vi "ParameterCtl.vi"(8 "error in":errorcluster caption="错误输入（无错误）", 9 "设备索引":u16(ring) caption="索引" items=["0", "1", "2", "3", "4", "5", "6", "7"], 11 "参数输入":T3={"帧ID1"=0, "等待延时"=0, "间隔延时"=0, "总时间"=0, "总次数"=0, "发送数据1"="", "接收数据1"="", "发送数据2"="", "接收数据2"="", "CAN盒类型"=3, "帧ID2"=0, "同步启动个数"=8, "模式"=enum."整体", "Baud"=12} {"Baud" items=["250k bps"=10, "10k bps"=2, "5k bps"=1, "50k bps"=5, "40k bps"=4, "20k bps"=3, "80k bps"=6, "100k bps"=7, "125k bps"=8, "200k bps"=9, "400k bps"=11, "500k bps"=12, "666k bps"=13, "800k bps"=14, "1000k bps"=15]; "帧ID2" format="%.0x"; "CAN盒类型" items=["PCI-CAN200"=7, "USB-CAN"=2, "USB-CAN200"=3]; "帧ID1" format="%.0x"}) -> (0 "error out":errorcluster caption="错误输出", 3 "输出":T2 {"DeviceType" items=["PCI-CAN200"=7, "USB-CAN"=2, "USB-CAN200"=3]})   [LabVIEW 2013]
uses:
  USBCAN/DevType.ctl
panel:
  # "ms"
  # "ms"
  # "s"
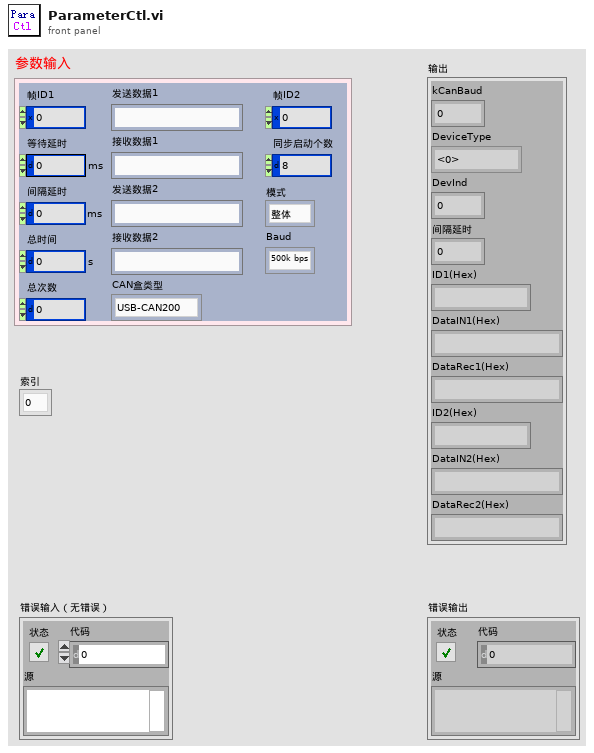
[diagram p1: front panel]
types:
  T1 = typedef "DevType.ctl" = u16
  T2 = cluster{"kCanBaud":u8, "DeviceType":T1, "DevInd":u16, "间隔延时":u32, "ID1(Hex)":string, "DataIN1(Hex)":string, "DataRec1(Hex)":string, "ID2(Hex)":string, "DataIN2(Hex)":string, "DataRec2(Hex)":string}
  T3 = cluster{"帧ID1":u32, "等待延时":u32, "间隔延时":u32, "总时间":u32, "总次数":u32, "发送数据1":string, "接收数据1":string, "发送数据2":string, "接收数据2":string, "CAN盒类型":T1, "帧ID2":u32, "同步启动个数":u8, "模式":enum16{"整体", "单个"}, "Baud":u8}
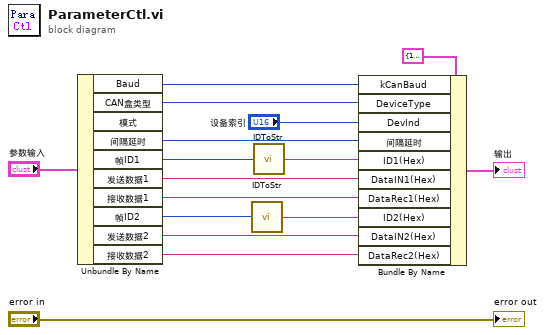
[diagram p0: block diagram]
diagram:
  n1 = Unbundle By Name("参数输入") -> ("Baud"=w14:u8, "CAN盒类型"=w13:T1, "间隔延时"=w12:u32, "帧ID1"=w5:u32, "发送数据1"=w11:string, "接收数据1"=w10:string, "帧ID2"=w3:u32, "发送数据2"=w9:string, "接收数据2"=w8:string)  [unwired: 1 out]
  n2 = call "IDToStr.vi"("帧ID输入"=w3) -> ("帧ID输出"=w2:string)
  n3 = call "IDToStr.vi"("帧ID输入"=w5) -> ("帧ID输出"=w4:string)
  n4 = Bundle By Name(cluster=T2 {"kCanBaud"=12, "DeviceType"=3, "DevInd"=0, "间隔延时"=0, "ID1(Hex)"="00000182", "DataIN1(Hex)"="000007d100000000", "DataRec1(Hex)"="000007d100000000", "ID2(Hex)"="00000182", "DataIN2(Hex)"="000007d100000000", "DataRec2(Hex)"="000007d100000000"} ("ParaIn"), "kCanBaud"=w14, "DeviceType"=w13, "DevInd"="设备索引", "间隔延时"=w12, "ID1(Hex)"=w4, "DataIN1(Hex)"=w11, "DataRec1(Hex)"=w10, "ID2(Hex)"=w2, "DataIN2(Hex)"=w9, "DataRec2(Hex)"=w8) -> (→"输出":T2)
  "error out" <- "error in"
